vi "Client Cancel Call.vi"(8 "error in":errorcluster, 11 "Call ID in":T1) -> (0 "error out":errorcluster, 1 "errorDetails":T2, 3 "Call ID out":T1)   [LabVIEW 2019, in "grpc-lvsupport.lvlib"]
uses:
  grpc-lvsupport.lvlib
  Shared/grpcId.ctl
  Shared/Any.ctl
  <vilib>/Utility/error.llb/Error Cluster From Error Code.vi
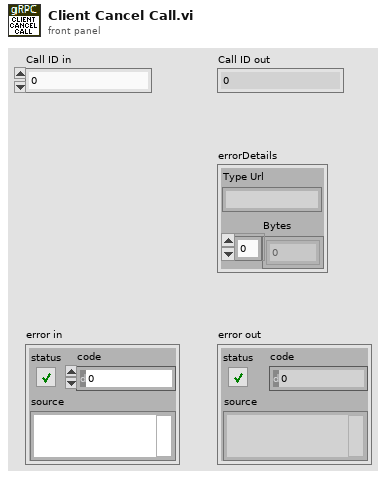
[diagram p1: front panel]
types:
  T1 = typedef "grpc-lvsupport.lvlib/grpcId.ctl" = u64
  T2 = typedef "grpc-lvsupport.lvlib/Any.ctl" = cluster{"Type Url":string, "Bytes":u8[]}
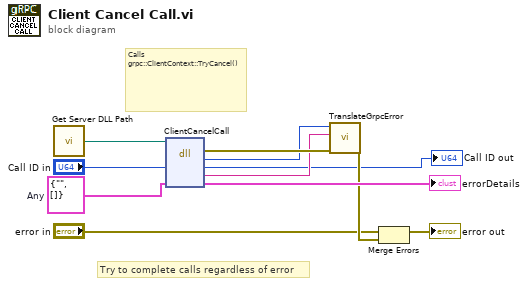
[diagram p0: block diagram]
diagram:
  w8 = T2 {"Type Url"="", "Bytes"=[]}  # Any
  # "Calls \ngrpc::ClientContext::TryCancel()"
  # "Try to complete calls regardless of error"
  n1 = call "Get Server DLL Path.vi"() -> ("server dll path"=w9:path)
  n2 = dll-call lib="?" fn="ClientCancelCall"(path in=w9, "ClientId"="Call ID in", "errorDetails"=w8) -> (error out=w11:errorcluster, "return type"=w5:i32, "ClientId"=→"Call ID out":u64, "errorMessage"=w6:string, "errorDetails"=→"errorDetails":T2)  [unwired: 3 in, 1 out]
  n3 = call "TranslateGrpcError.vi"("error in"=w11, "Error Message"=w6, "Error Code"=w5) -> ("error out"=w4:errorcluster)  [unwired: 8 in]
  n4 = Merge Errors("error in", w4) -> (→"error out":errorcluster)
